vi "Initialize.vi"(8 "error in":errorcluster, 10 "Session":string="TSI 3550", 11 "Neph In":refnum<class "Nephelometer.lvclass">) -> (0 "error out":errorcluster, 3 "Neph Out":refnum<class "Nephelometer.lvclass">)   [LabVIEW 2014, in "Nephelometer.lvclass"]
uses:
  Nephelometer.lvclass
  Reusable/Session APIs/Serial/Serial Session.lvclass
  Reusable/Session APIs/File Access/Config Data/Config Data.lvclass
  Configurable Device/Configurable Device.lvclass/Configurable Device.ctl
  Reusable/Session APIs/File Access/Config Data/Config Data.lvclass/Config Data.ctl
  Nephelometer.lvclass/Nephelometer.ctl
  Configurable Device/Read Handle.vi
  Reusable/Session APIs/File Access/Config Data/Accessors/Read Cfg Path.vi
  Reusable/Session APIs/File Access/Config Data/Accessors/Write Cfg Path.vi
  Reusable/Session APIs/File Access/Config Data/Accessors/Read Ref.vi
  Accessors/Write Session Handle.vi
  <userlib>/_Session Fwk/Accessors/_get Session Name for PN.vi
  <vilib>/Utility/config.llb/Read Key (U32).vi
  Unpolled Commands/Power.vi
  Unpolled Commands/Start_Stop Polling Mode.vi
  Unpolled Commands/Set Blower Level.vi
  Unpolled Commands/Set Blank Time.vi
  Unpolled Commands/Set Autozero Time.vi
  Unpolled Commands/Set Autozero Period.vi
  Unpolled Commands/Set Zero Mode.vi
  <vilib>/Utility/config.llb/NI_LVConfig.lvlib
  <userlib>/_Session Fwk/Session - Root.lvclass
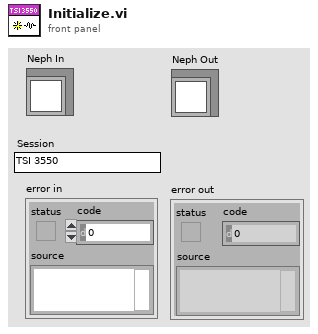
[diagram p1: front panel]
types:
  T1 = typedef "Config Data.lvclass/Config Session.ctl" = refnum<data-value>
  T2 = typedef "Session - Root.lvclass/Session Handle.ctl" = refnum<data-value>
  T3 = typedef "NI_LVConfig.lvlib/Config Data RefNum.ctl" = refnum<k1>
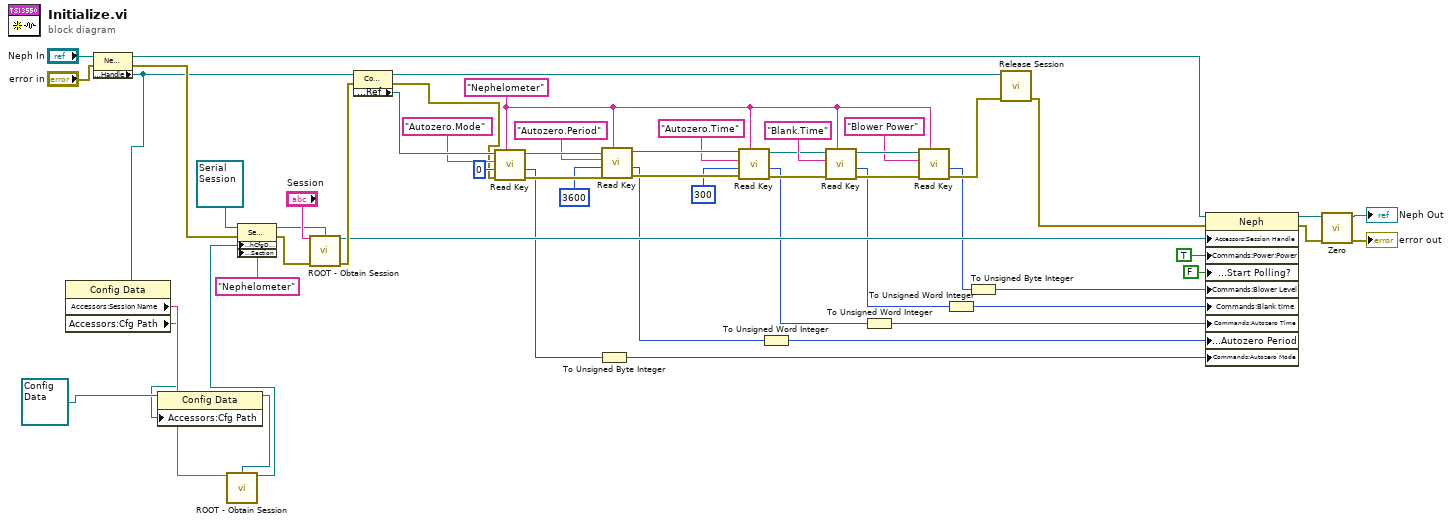
[diagram p0: block diagram]
diagram:
  w35 = "Nephelometer" ("Section Name")
  n1 = property class="Neph"(reference="Neph In", error in="error in") -> (reference out=w19:refnum<class "Nephelometer.lvclass">, error out=w22:errorcluster, "Accessors:Handle"=w6:T1)
  n2 = property class="Config Data"(reference=w6) -> ("Accessors:Session Name"=w5:string, "Accessors:Cfg Path"=w3:path)  [unwired: 1 in, 2 out]
  n3 = property class="Config Data"(reference=refnum<class "Config Data.lvclass"> refnum ("Config Data"), "Accessors:Cfg Path"=w3) -> (reference out=w2:refnum<class "Config Data.lvclass">)  [unwired: 1 in, 1 out]
  n4 = call <userlib>:"ROOT - Obtain Session.vi"("Session Name ()"=w5, "OBJ - Session"=w2) -> ("Session Handle"=w1:T2)  [unwired: 11 in, 2 out]
  n5 = property class="Serial Session"(reference=refnum<class "Serial Session.lvclass"> refnum ("Serial Session in"), error in=w22, "Accessors:hCfgData"=w1, "Accessors:Section"="Nephelometer" ("Section Name")) -> (reference out=w24:refnum<class "Serial Session.lvclass">, error out=w21:errorcluster)
  n6 = call <userlib>:"ROOT - Obtain Session.vi"("Session Name ()"="Session", "OBJ - Session"=w24, "error in (no error)"=w21) -> ("Session Handle"=w18:T2, "error out"=w20:errorcluster)  [unwired: 10 in, 1 out]
  n7 = property class="Config Data"(reference=w6, error in=w20) -> (reference out=w54:T1, error out=w7:errorcluster, "Accessors:Ref"=w53:T3)
  n8 = call-poly <vilib>:"Read Key.vi"("section"=w35, "error in (no error)"=w7, "default value"=u32 0, "key"="Autozero.Mode", "refnum"=w53) -> ("error out"=w50:errorcluster, "value"=w10:u32, "refnum out"=w51:T3)  [unwired: 3 in, 1 out]
  n9 = To Unsigned Byte Integer(number=w10) -> (unsigned 8bit integer=w9:u8)
  n10 = call-poly <vilib>:"Read Key.vi"("section"=w35, "error in (no error)"=w50, "default value"=u32 3600, "key"="Autozero.Period", "refnum"=w51) -> ("error out"=w40:errorcluster, "value"=w12:u32, "refnum out"=w41:T3)  [unwired: 3 in, 1 out]
  n11 = call-poly <vilib>:"Read Key.vi"("section"=w35, "error in (no error)"=w40, "default value"=u32 300, "key"="Autozero.Time", "refnum"=w41) -> ("error out"=w36:errorcluster, "value"=w15:u32, "refnum out"=w37:T3)  [unwired: 3 in, 1 out]
  n12 = To Unsigned Word Integer(number=w12) -> (unsigned 16bit integer=w11:u16)
  n13 = call-poly <vilib>:"Read Key.vi"("section"=w35, "error in (no error)"=w36, "key"="Blank.Time", "refnum"=w37) -> ("error out"=w46:errorcluster, "value"=w14:u32, "refnum out"=w47:T3)  [unwired: 4 in, 1 out]
  n14 = To Unsigned Word Integer(number=w15) -> (unsigned 16bit integer=w8:u16)
  n15 = call-poly <vilib>:"Read Key.vi"("section"=w35, "error in (no error)"=w46, "key"="Blower Power", "refnum"=w47) -> ("error out"=w44:errorcluster, "value"=w17:u32)  [unwired: 4 in, 2 out]
  n16 = To Unsigned Word Integer(number=w14) -> (unsigned 16bit integer=w13:u16)
  n17 = To Unsigned Byte Integer(number=w17) -> (unsigned 8bit integer=w16:u8)
  n18 = call "Release Session.vi"("error in"=w44, "Session Handle"=w54) -> ("error out"=w31:errorcluster)  [unwired: 8 in, 1 out]
  n19 = property class="Neph"(reference=w19, error in=w31, "Accessors:Session Handle"=w18, "Commands:Power:Power"=TRUE ("Power"), "Commands:Polling:Start Polling?"=FALSE ("Start Polling?"), "Commands:Blower Level"=w16, "Commands:Blank time"=w13, "Commands:Autozero Time"=w8, "Commands:Autozero Period"=w11, "Commands:Autozero Mode"=w9) -> (reference out=w34:refnum<class "Nephelometer.lvclass">, error out=w32:errorcluster)
  n20 = call "Zero.vi"("error in"=w32, "Neph in"=w34) -> ("error out"=→"error out":errorcluster, "Neph out"=→"Neph Out":refnum<class "Nephelometer.lvclass">)  [unwired: 8 in]
